vi "Read ADCs.vi"   [LabVIEW 2018]
uses:
  MCP3008/MCP3008.lvlib
  MCP3008/Configuration Bits.ctl
  <vilib>/rvi/DataTransferAndStorage/Container/XNode/niFpgaContainer.xnode
  <vilib>/rvi/interface/RandomDataEmulation/nirviRandomDataFpgaReadWriteTemplate.vi
types:
  T1 = typedef "MCP3008.lvlib/Configuration Bits.ctl" = u8
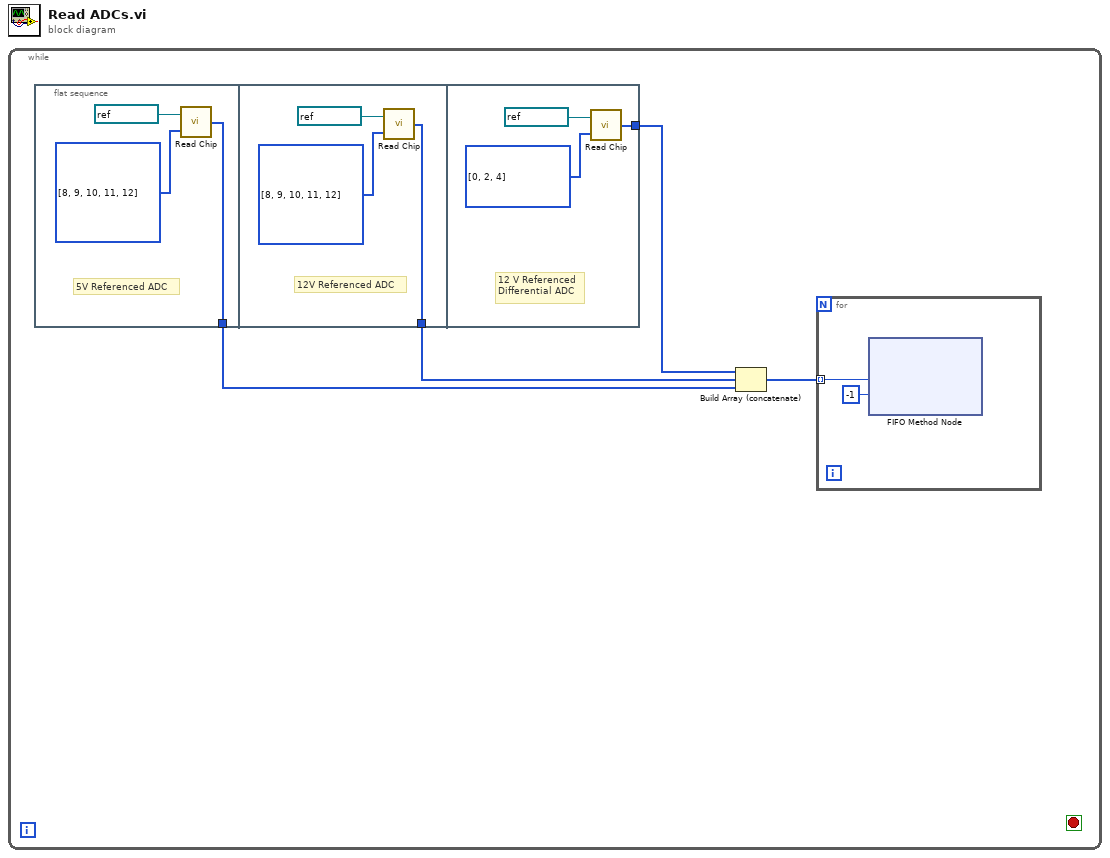
[diagram p0: block diagram]
diagram:
  n1 = while {
    stop <- _ stop-if-true
    n2 = flat-sequence {
      tunnel: [w5] -> w2
      tunnel: [w8] -> w3
      tunnel: [w11] -> w4
      frame #0 {
        w6 = T1[] [8, 9, 10, 11, 12] items=["Ch 0 SE"=8, "Ch 1 SE"=9, "Ch 2 SE"=10, "Ch 3 SE"=11, "Ch 4 SE"=12, "Ch 5 SE"=13, "Ch 6 SE"=14, "Ch 7 SE"=15, "Diff 0+ 1-"=0, "Diff 1+ 0-"=1, "Diff 2+ 3-"=2, "Diff 3+ 2-"=3, "Diff 4+ 5-"=4, "Diff 5+ 4-"=5, "Diff 6+ 7-"=6, "Diff 7+ 6-"=7] ("Config Bits")
        # "5V Referenced ADC"
        n3 = call "Read Chip.vi"("Config Bits"=w6, "ADC CS line"=refnum<k21> "AI_CS1") -> ("Read Values"=w5:u16[])
      }
      frame #1 {
        w10 = T1[] [8, 9, 10, 11, 12] items=["Ch 0 SE"=8, "Ch 1 SE"=9, "Ch 2 SE"=10, "Ch 3 SE"=11, "Ch 4 SE"=12, "Ch 5 SE"=13, "Ch 6 SE"=14, "Ch 7 SE"=15, "Diff 0+ 1-"=0, "Diff 1+ 0-"=1, "Diff 2+ 3-"=2, "Diff 3+ 2-"=3, "Diff 4+ 5-"=4, "Diff 5+ 4-"=5, "Diff 6+ 7-"=6, "Diff 7+ 6-"=7] ("Config Bits")
        # "12V Referenced ADC"
        n4 = call "Read Chip.vi"("Config Bits"=w10, "ADC CS line"=refnum<k21> "AI_CS2") -> ("Read Values"=w8:u16[])
      }
      frame #2 {
        w12 = T1[] [0, 2, 4] items=["Ch 0 SE"=8, "Ch 1 SE"=9, "Ch 2 SE"=10, "Ch 3 SE"=11, "Ch 4 SE"=12, "Ch 5 SE"=13, "Ch 6 SE"=14, "Ch 7 SE"=15, "Diff 0+ 1-"=0, "Diff 1+ 0-"=1, "Diff 2+ 3-"=2, "Diff 3+ 2-"=3, "Diff 4+ 5-"=4, "Diff 5+ 4-"=5, "Diff 6+ 7-"=6, "Diff 7+ 6-"=7] ("Config Bits")
        # "12 V Referenced\nDifferential ADC"
        n5 = call "Read Chip.vi"("Config Bits"=w12, "ADC CS line"=refnum<k21> "AI_CS3") -> ("Read Values"=w11:u16[])
      }
    }
    n6 = Build Array (concatenate)(w4, w3, w2) -> (w1:u16[])
    n7 = for {
      tunnel: w1 -> [w15] mode=indexing
      n8 = xnode ("FIFO Method Node")("Element"=w15, "Timeout"=-1) -> ()  [unwired: 1 in, 2 out]
    }
  }
